vi "Delete RPC VI Template.vi"(8 "error in (no error)":errorcluster, 11 "LVClassLibrary in":refnum<vi>) -> (0 "error out":errorcluster, 3 "LVClassLibrary out":refnum<vi>)   [LabVIEW 2019, in "gRPC Template Creation Utility.lvlib"]
uses:
  gRPC Template Creation Utility.lvlib
  ServiceConstants.ctl
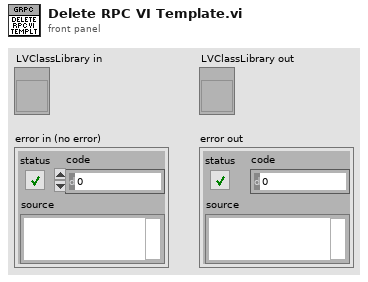
[diagram p1: front panel]
types:
  T1 = typedef "gRPC Template Creation Utility.lvlib/ServiceConstants.ctl" = enum16{"Stub", "Impl", "Usercode_server", "Generated_server", "RPC Service", "RPC Method package_service_method", "ServiceClass out", "ServiceClass in", "RPC Method"}
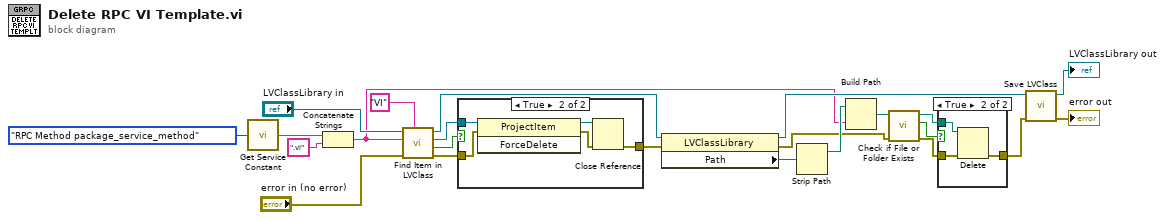
[diagram p0: block diagram]
diagram:
  n1 = call "Get Service Constant.vi"("Service Constant Strings"=ServiceConstants."RPC Method package_service_method") -> ("String Value"=w20:string)
  n2 = Concatenate Strings(w20, ".vi" ("string")) -> (w8:string)
  n3 = call "Find Item in LVClass.vi"("Item Type"="VI", "error in (no error)"="error in (no error)", "Item Name"=w8, "Class Item in"="LVClassLibrary in") -> ("error out"=w14:errorcluster, "Found?"=w13:bool, "Project Item (Class Item)"=w15:refnum<vi>, "Class Item out"=w12:refnum<vi>)  [unwired: 4 in]
  n4 = case shown="True" w13 {
    tunnel: w15 -> [_ w26]
    tunnel: w14 -> [w24 w25]
    tunnel: [w24 w27] -> w3
    frame False {
    }
    frame True {
      n5 = invoke class="ProjectItem" method="ForceDelete"(reference=w26, error in=w25) -> (reference out=w28:refnum<vi>, error out=w29:errorcluster)  [unwired: 1 in, 1 out]
      n6 = Close Reference(reference=w28, error in (no error)=w29) -> (error out=w27:errorcluster)
    }
  }
  n7 = property class="LVClassLibrary"(reference=w12, error in=w3) -> (reference out=w11:refnum<vi>, error out=w2:errorcluster, "Path"=w10:path)
  n8 = Strip Path(path=w10) -> (stripped path=w9:path)  [unwired: 1 out]
  n9 = Build Path(base path=w9, name or relative path=w8) -> (appended path=w7:path)
  n10 = call <vilib>:"Check if File or Folder Exists.vi"("error in (no error)"=w2, "path"=w7) -> ("error out"=w4:errorcluster, "file or folder exists?"=w5:bool, "dup path"=w6:path)  [unwired: 7 in]
  n11 = case shown="True" w5 {
    tunnel: w6 -> [_ w33]
    tunnel: w4 -> [w30 w32]
    tunnel: [w30 w31] -> w1
    frame False {
    }
    frame True {
      n12 = Delete(path (use dialog)=w33, error in=w32) -> (error out=w31:errorcluster)  [unwired: 3 in, 2 out]
    }
  }
  n13 = call "Save LVClass.vi"("error in (no error)"=w1, "LVClassLibrary in"=w11) -> ("error out"=→"error out":errorcluster, "LVClassLibrary out"=→"LVClassLibrary out":refnum<vi>)  [unwired: 8 in]
